vi "RoboticArm.vi"() -> ()   [LabVIEW 2018]
uses:
  <vilib>/LabVIEW Interface for Arduino/Type Defs/Board Type.ctl
  <vilib>/LabVIEW Interface for Arduino/Type Defs/Connection Type.ctl
  <vilib>/LabVIEW Interface for Arduino/LabVIEW Interface for Arduino.lvlib
panel:
  in  "Arm 2":i32(slide) scale=-360.0..360.0
  in  "MOTION 3":bool
  in  "Arm1":i32(slide) scale=-360.0..360.0
  in  "MOTION 2":bool
  in  "Height":i32(slide) scale=-10.0..10.0
  in  "M2":bool
  in  "Base Rotation":i32(slide) scale=-360.0..360.0
  in  "STOP MOTION":bool
  in  "Start Arm\nMovement":bool
  in  "MOTION":bool
  in  "Gripper Angle (Degrees)":u8(knob)=15 scale=0.0..180.0
  out "Error":errorcluster
  in  "Baud Rate":u32=115200
  in  "Board Type (Uno)":T1
  in  "VISA resource":refnum<visa-resource-name>
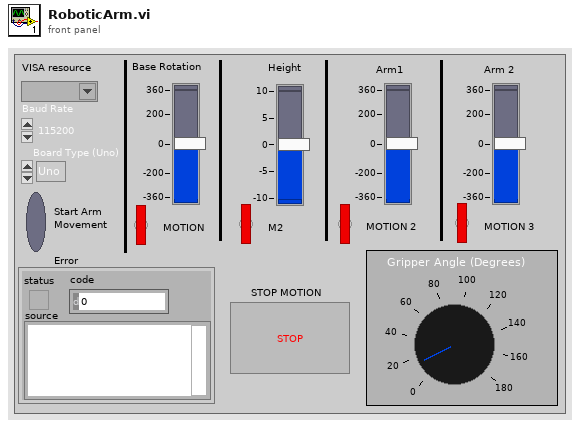
[diagram p1: front panel]
types:
  T1 = typedef "LabVIEW Interface for Arduino.lvlib/Board Type.ctl" = enum16{"Uno", "Dimuelanove w/Atmega 328", "Mega 2560"}
  T2 = typedef "LabVIEW Interface for Arduino.lvlib/Connection Type.ctl" = enum8{"USB / Serial", "XBEE", "BlueSmirf (Bluetooth)"}
  T3 = typedef "LabVIEW Interface for Arduino.lvlib/Arduino Resource.ctl" = cluster{"VISA resource":refnum<visa-resource-name>, "Board Type":T1, "Connection Type":enum8{"USB / Serial"}, "Bytes Per Packet (15)":u8}
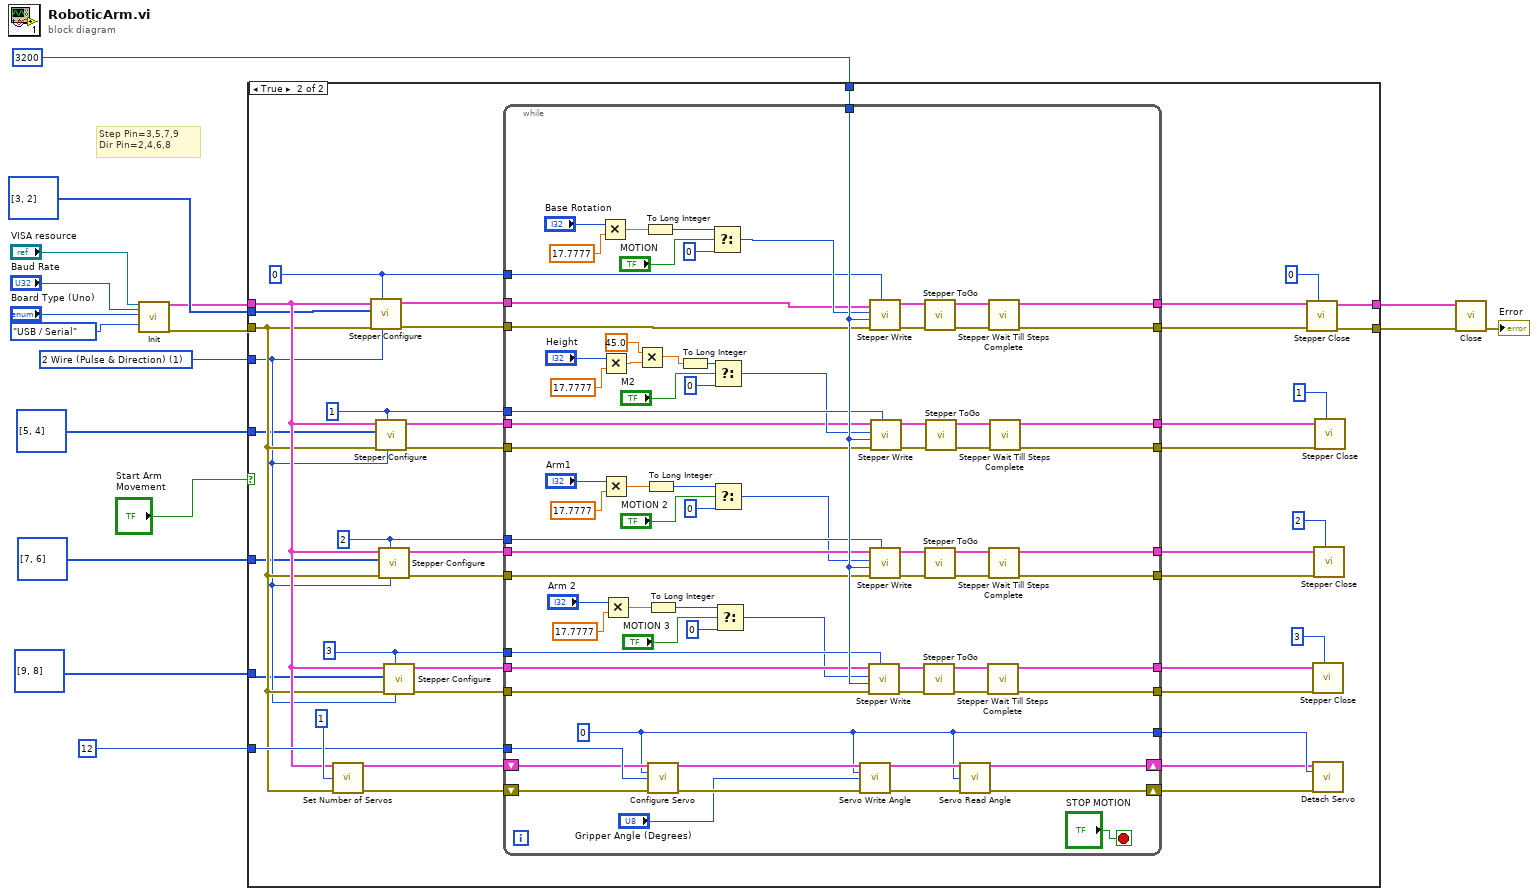
[diagram p0: block diagram]
diagram:
  w4 = u8 1 items=["2 Wire (Pulse & Direction)"=1, "2 Wire"=2, "4 Wire"=4, "EasyDriver"=6, "AF Motor Shield (Stepper 1 & 2 Only)"=5] ("Control Method")
  # "Step Pin=3,5,7,9\nDir Pin=2,4,6,8"
  n1 = call <vilib>:"Init.vi"("VISA resource"="VISA resource", "Baud Rate (115200)"="Baud Rate", "Board Type (Uno)"="Board Type (Uno)", "Connection Type (USB/Serial)"=Connection_Type."USB / Serial") -> ("Arduino Resource"=w10:T3, "error out"=w9:errorcluster)  [unwired: 14 in]
  n2 = case shown="True" "Start Arm\nMovement" {
    tunnel: u8[] [3, 2] ("Stepper Pins") -> [_ w37]
    tunnel: u8 12 ("DIO Pin (2)") -> [_ w59]
    tunnel: w10 -> [w19 w40]
    tunnel: w9 -> [w18 w39]
    tunnel: u8[] [5, 4] ("Stepper Pins") -> [_ w34]
    tunnel: u8[] [7, 6] ("Stepper Pins") -> [_ w31]
    tunnel: u8[] [9, 8] ("Stepper Pins") -> [_ w28]
    tunnel: i16 3200 ("Set Speed (Steps per Second)") -> [_ w56]
    tunnel: w4 -> [_ w38]
    tunnel: [w19 w43] -> w2
    tunnel: [w18 w42] -> w1
    frame False {
    }
    frame True {
      w53 = u8 3 ("Stepper #")
      w55 = u8 2 ("Stepper #")
      w54 = u8 1 ("Stepper #")
      w41 = u8 0 ("Stepper #")
      n3 = call <vilib>:"Set Number of Servos.vi"("Arduino Resource"=w40, "Number Of Servos (1)"=u8 1, "error in"=w39) -> ("Arduino Resource"=w58:T3, "error out"=w57:errorcluster)  [unwired: 11 in]
      n4 = call <vilib>:"Stepper Configure.vi"("Control Method"=w38, "Stepper #"=w41, "error in"=w39, "Stepper Pins"=w37, "Arduino Resource"=w40) -> ("error out"=w36:errorcluster, "Arduino Resource Out"=w35:T3)  [unwired: 5 in]
      n5 = call <vilib>:"Stepper Configure.vi"("Control Method"=w38, "Stepper #"=w54, "error in"=w39, "Stepper Pins"=w34, "Arduino Resource"=w40) -> ("error out"=w33:errorcluster, "Arduino Resource Out"=w32:T3)  [unwired: 5 in]
      n6 = call <vilib>:"Stepper Configure.vi"("Control Method"=w38, "Stepper #"=w55, "error in"=w39, "Stepper Pins"=w31, "Arduino Resource"=w40) -> ("error out"=w30:errorcluster, "Arduino Resource Out"=w29:T3)  [unwired: 5 in]
      n7 = call <vilib>:"Stepper Configure.vi"("Control Method"=w38, "Stepper #"=w53, "error in"=w39, "Stepper Pins"=w28, "Arduino Resource"=w40) -> ("error out"=w27:errorcluster, "Arduino Resource Out"=w26:T3)  [unwired: 5 in]
      n8 = while {
        tunnel: w59 -> [w135]
        tunnel: w56 -> [w115]
        tunnel: w55 -> [w114]
        tunnel: w54 -> [w113]
        tunnel: w53 -> [w112]
        tunnel: [w111] -> w52
        tunnel: [w107] -> w49
        tunnel: [w106] -> w48
        tunnel: [w105] -> w47
        tunnel: [w104] -> w46
        tunnel: [w103] -> w45
        tunnel: [w102] -> w44
        tunnel: w41 -> [w101]
        shift-right: [w109] -> w51
        shift-left: w58 -> [w129]
        shift-right: [w108] -> w50
        shift-left: w57 -> [w128]
        tunnel: w36 -> [w98]
        tunnel: w35 -> [w97]
        tunnel: w33 -> [w85]
        tunnel: w32 -> [w84]
        tunnel: w30 -> [w83]
        tunnel: w29 -> [w82]
        tunnel: w27 -> [w81]
        tunnel: w26 -> [w80]
        tunnel: [w79] -> w25
        tunnel: [w78] -> w24
        stop <- "STOP MOTION" stop-if-true
        w111 = u8 0 ("Servo Number (0)")
        n9 = Multiply(x="Base Rotation", y=17.7777) -> (x*y=w92:dbl)
        n10 = Multiply(x="Height", y=17.7777) -> (x*y=w87:dbl)
        n11 = Multiply(x="Arm1", y=17.7777) -> (x*y=w72:dbl)
        n12 = Multiply(x="Arm 2", y=17.7777) -> (x*y=w65:dbl)
        n13 = Multiply(x=45.0, y=w87) -> (x*y=w63:dbl)
        n14 = To Long Integer(number=w92) -> (32bit integer=w94:i32)
        n15 = To Long Integer(number=w72) -> (32bit integer=w74:i32)
        n16 = To Long Integer(number=w65) -> (32bit integer=w67:i32)
        n17 = call <vilib>:"Configure Servo.vi"("Arduino Resource"=w129, "Servo Number (0)"=w111, "DIO Pin (2)"=w135, "error in"=w128) -> ("Arduino Resource"=w134:T3, "error out"=w133:errorcluster)  [unwired: 10 in]
        n18 = To Long Integer(number=w63) -> (32bit integer=w89:i32)
        n19 = Select(t=w94, s="MOTION", f=0) -> (s? t:f=w110:i32)
        n20 = Select(t=w89, s="M2", f=0) -> (s? t:f=w86:i32)
        n21 = Select(t=w74, s="MOTION 2", f=0) -> (s? t:f=w71:i32)
        n22 = Select(t=w67, s="MOTION 3", f=0) -> (s? t:f=w64:i32)
        n23 = call <vilib>:"Servo Write Angle.vi"("Arduino Resource"=w134, "Servo Number"=w111, "Angle (Degrees)"="Gripper Angle (Degrees)", "error in"=w133) -> ("Arduino Resource"=w131:T3, "error out"=w130:errorcluster)  [unwired: 10 in]
        n24 = call <vilib>:"Stepper Write.vi"("Stepper #"=w112, "error in"=w81, "Set Speed (Steps per Second)"=w115, "# of Steps to Move"=w64, "Arduino Resource"=w80) -> ("error out"=w118:errorcluster, "Arduino Resource Out"=w119:T3)  [unwired: 5 in]
        n25 = call <vilib>:"Stepper Write.vi"("Stepper #"=w101, "error in"=w98, "Set Speed (Steps per Second)"=w115, "# of Steps to Move"=w110, "Arduino Resource"=w97) -> ("error out"=w137:errorcluster, "Arduino Resource Out"=w139:T3)  [unwired: 5 in]
        n26 = call <vilib>:"Stepper Write.vi"("Stepper #"=w114, "error in"=w83, "Set Speed (Steps per Second)"=w115, "# of Steps to Move"=w71, "Arduino Resource"=w82) -> ("error out"=w121:errorcluster, "Arduino Resource Out"=w123:T3)  [unwired: 5 in]
        n27 = call <vilib>:"Stepper Write.vi"("Stepper #"=w113, "error in"=w85, "Set Speed (Steps per Second)"=w115, "# of Steps to Move"=w86, "Arduino Resource"=w84) -> ("error out"=w125:errorcluster, "Arduino Resource Out"=w127:T3)  [unwired: 5 in]
        n28 = call <vilib>:"Stepper ToGo.vi"("error in"=w118, "Arduino Resource"=w119) -> ("error out"=w116:errorcluster, "Arduino Resource Out"=w117:T3)  [unwired: 6 in, 2 out]
        n29 = call <vilib>:"Stepper ToGo.vi"("error in"=w137, "Arduino Resource"=w139) -> ("error out"=w136:errorcluster, "Arduino Resource Out"=w138:T3)  [unwired: 6 in, 2 out]
        n30 = call <vilib>:"Stepper ToGo.vi"("error in"=w121, "Arduino Resource"=w123) -> ("error out"=w120:errorcluster, "Arduino Resource Out"=w122:T3)  [unwired: 6 in, 2 out]
        n31 = call <vilib>:"Stepper ToGo.vi"("error in"=w125, "Arduino Resource"=w127) -> ("error out"=w124:errorcluster, "Arduino Resource Out"=w126:T3)  [unwired: 6 in, 2 out]
        n32 = call <vilib>:"Servo Read Angle.vi"("Arduino Resource"=w131, "Servo Number"=w111, "error in"=w130) -> ("Arduino Resource"=w109:T3, "error out"=w108:errorcluster)  [unwired: 10 in, 1 out]
        n33 = call <vilib>:"Stepper Wait Till Steps Complete.vi"("error in"=w116, "Arduino Resource In"=w117) -> ("error out"=w107:errorcluster, "Arduino Resource Out"=w106:T3)  [unwired: 8 in]
        n34 = call <vilib>:"Stepper Wait Till Steps Complete.vi"("error in"=w136, "Arduino Resource In"=w138) -> ("error out"=w102:errorcluster, "Arduino Resource Out"=w103:T3)  [unwired: 8 in]
        n35 = call <vilib>:"Stepper Wait Till Steps Complete.vi"("error in"=w120, "Arduino Resource In"=w122) -> ("error out"=w105:errorcluster, "Arduino Resource Out"=w104:T3)  [unwired: 8 in]
        n36 = call <vilib>:"Stepper Wait Till Steps Complete.vi"("error in"=w124, "Arduino Resource In"=w126) -> ("error out"=w78:errorcluster, "Arduino Resource Out"=w79:T3)  [unwired: 8 in]
      }
      n37 = call <vilib>:"Stepper Close.vi"("Stepper #"=u8 0, "error in"=w44, "Arduino Resource"=w45) -> ("error out"=w42:errorcluster, "Arduino Resource Out"=w43:T3)  [unwired: 7 in]
      n38 = call <vilib>:"Stepper Close.vi"("Stepper #"=u8 3, "error in"=w49, "Arduino Resource"=w48) -> ()  [unwired: 7 in, 2 out]
      n39 = call <vilib>:"Detach Servo.vi"("Arduino Resource"=w51, "Servo Number"=w52, "error in"=w50) -> ()  [unwired: 11 in, 2 out]
      n40 = call <vilib>:"Stepper Close.vi"("Stepper #"=u8 2, "error in"=w47, "Arduino Resource"=w46) -> ()  [unwired: 7 in, 2 out]
      n41 = call <vilib>:"Stepper Close.vi"("Stepper #"=u8 1, "error in"=w24, "Arduino Resource"=w25) -> ()  [unwired: 7 in, 2 out]
    }
  }
  n42 = call <vilib>:"Close.vi"("Arduino Resource"=w2, "error in"=w1) -> ("error out"=→"Error":errorcluster)  [unwired: 13 in]
